vi "Side_Height.vi"(8 "cos_theta":dbl, 9 "sin_theta":dbl, 10 "W":dbl format="%#_13g", 11 "H'":dbl format="%#_13g") -> (3 "H":dbl)   [LabVIEW 2019, in "Algorithm.lvclass"]
uses:
  FrameworkOverrides/Algorithm.lvclass
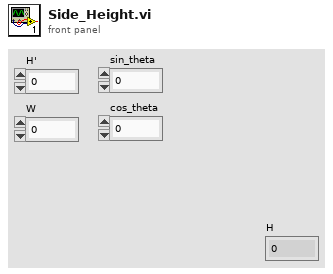
[diagram p1: front panel]
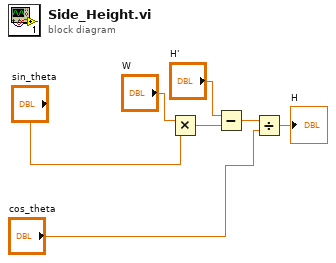
[diagram p0: block diagram]
diagram:
  n1 = Multiply(x="W", y="sin_theta") -> (x*y=w5:dbl)
  n2 = Subtract(x="H'", y=w5) -> (x-y=w4:dbl)
  n3 = Divide(x=w4, y="cos_theta") -> (x/y=→"H":dbl)
